vi "Set Package License.vi"(8 "error in (no error)":errorcluster, 10 "License":string, 11 "GPack File in":refnum<class "GPack File.lvclass">) -> (0 "error out":errorcluster, 3 "GPack File out":refnum<class "GPack File.lvclass">)   [LabVIEW 2020, in "GPack.lvlib" / "GPack File.lvclass"]
uses:
  GPack File.lvclass
  GPack File.lvclass/GPack File.ctl
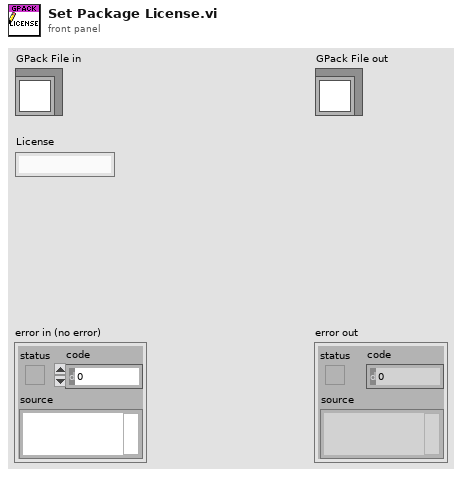
[diagram p1: front panel]
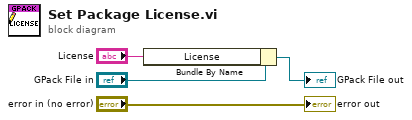
[diagram p0: block diagram]
diagram:
  n1 = Bundle By Name(cluster="GPack File in", "License"="License") -> (→"GPack File out":refnum<class "GPack File.lvclass">)
  "error out" <- "error in (no error)"
